vi "Unit test title.vi"(8 "error in (no error)":errorcluster, 11 "serializer":refnum<class "BlueSerializer.lvclass">) -> (0 "error out":errorcluster, 3 "Caraya test  label":string)   [LabVIEW 2019, in "Sports Unit Tests.lvclass"]
uses:
  Sports Unit Tests.lvclass
  <userlib>/Blue Origin/BlueSerialization/BlueSerializer/BlueSerializer.lvclass
  <vilib>/addons/_JKI Toolkits/Caraya/classes/Test/Test.lvclass
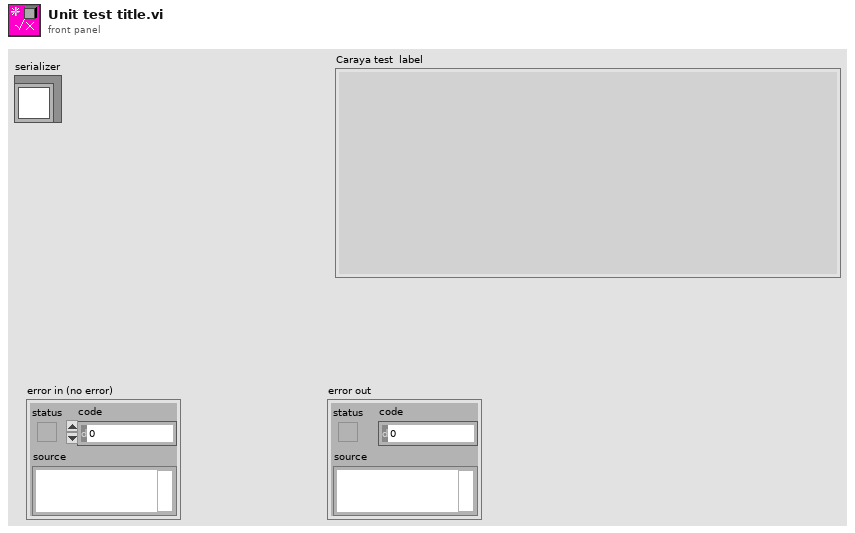
[diagram p1: front panel]
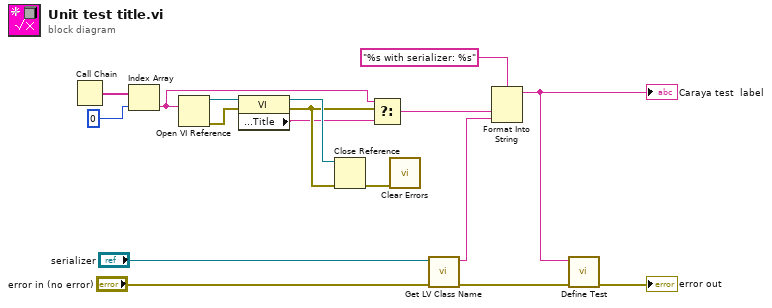
[diagram p0: block diagram]
diagram:
  n1 = Call Chain() -> (call chain=w13:string[])
  n2 = Index Array(array=w13, index=0 ("Level (1)")) -> (element=w11:string)
  n3 = Open VI Reference(vi path=w11) -> (vi reference=w16:refnum<vi>, error out=w15:errorcluster)  [unwired: 5 in]
  n4 = property class="VI"(reference=w16, error in=w15) -> (reference out=w14:refnum<vi>, error out=w12:errorcluster, "Front Panel Window:Title"=w10:string)
  n5 = Close Reference(reference=w14, error in (no error)=w12) -> (error out=w6:errorcluster)
  n6 = Select(t=w11, s=w12, f=w10) -> (s? t:f=w8:string)
  n7 = call <vilib>:"Clear Errors.vi"("error in (no error)"=w6) -> ()  [unwired: 5 in, 2 out]
  n8 = call <vilib>:"Get LV Class Name.vi"("error in (no error)"="error in (no error)", "object"="serializer") -> ("error out"=w2:errorcluster, "class name"=w7:string)  [unwired: 8 in]
  n9 = Format Into String(format string="%s with serializer: %s", w8, w7) -> (resulting string=w3:string)  [unwired: 2 in, 1 out]
  "Caraya test  label" <- w3
  n10 = call <vilib>:"Define Test.vi"("error in (no error)"=w2, "Label (VI Title)"=w3) -> ("error out"=→"error out":errorcluster)  [unwired: 9 in]
